vi "Conversor_4dados.vi"(2 "subarray":u8[](array[numeric])) -> (3 "ROCOF":sgl format="%_8g", 4 "Frequência":sgl format="%_8g", 5 "Ângulo":sgl format="%_8g", 6 "Módulo":sgl format="%_8g")   [LabVIEW 2018]
panel:
  out "sinal 4":bool
  out "sinal 3":bool
  out "sinal 2":bool
  out "sinal":bool
  # "Conversor de dados da serial - quadruplo"
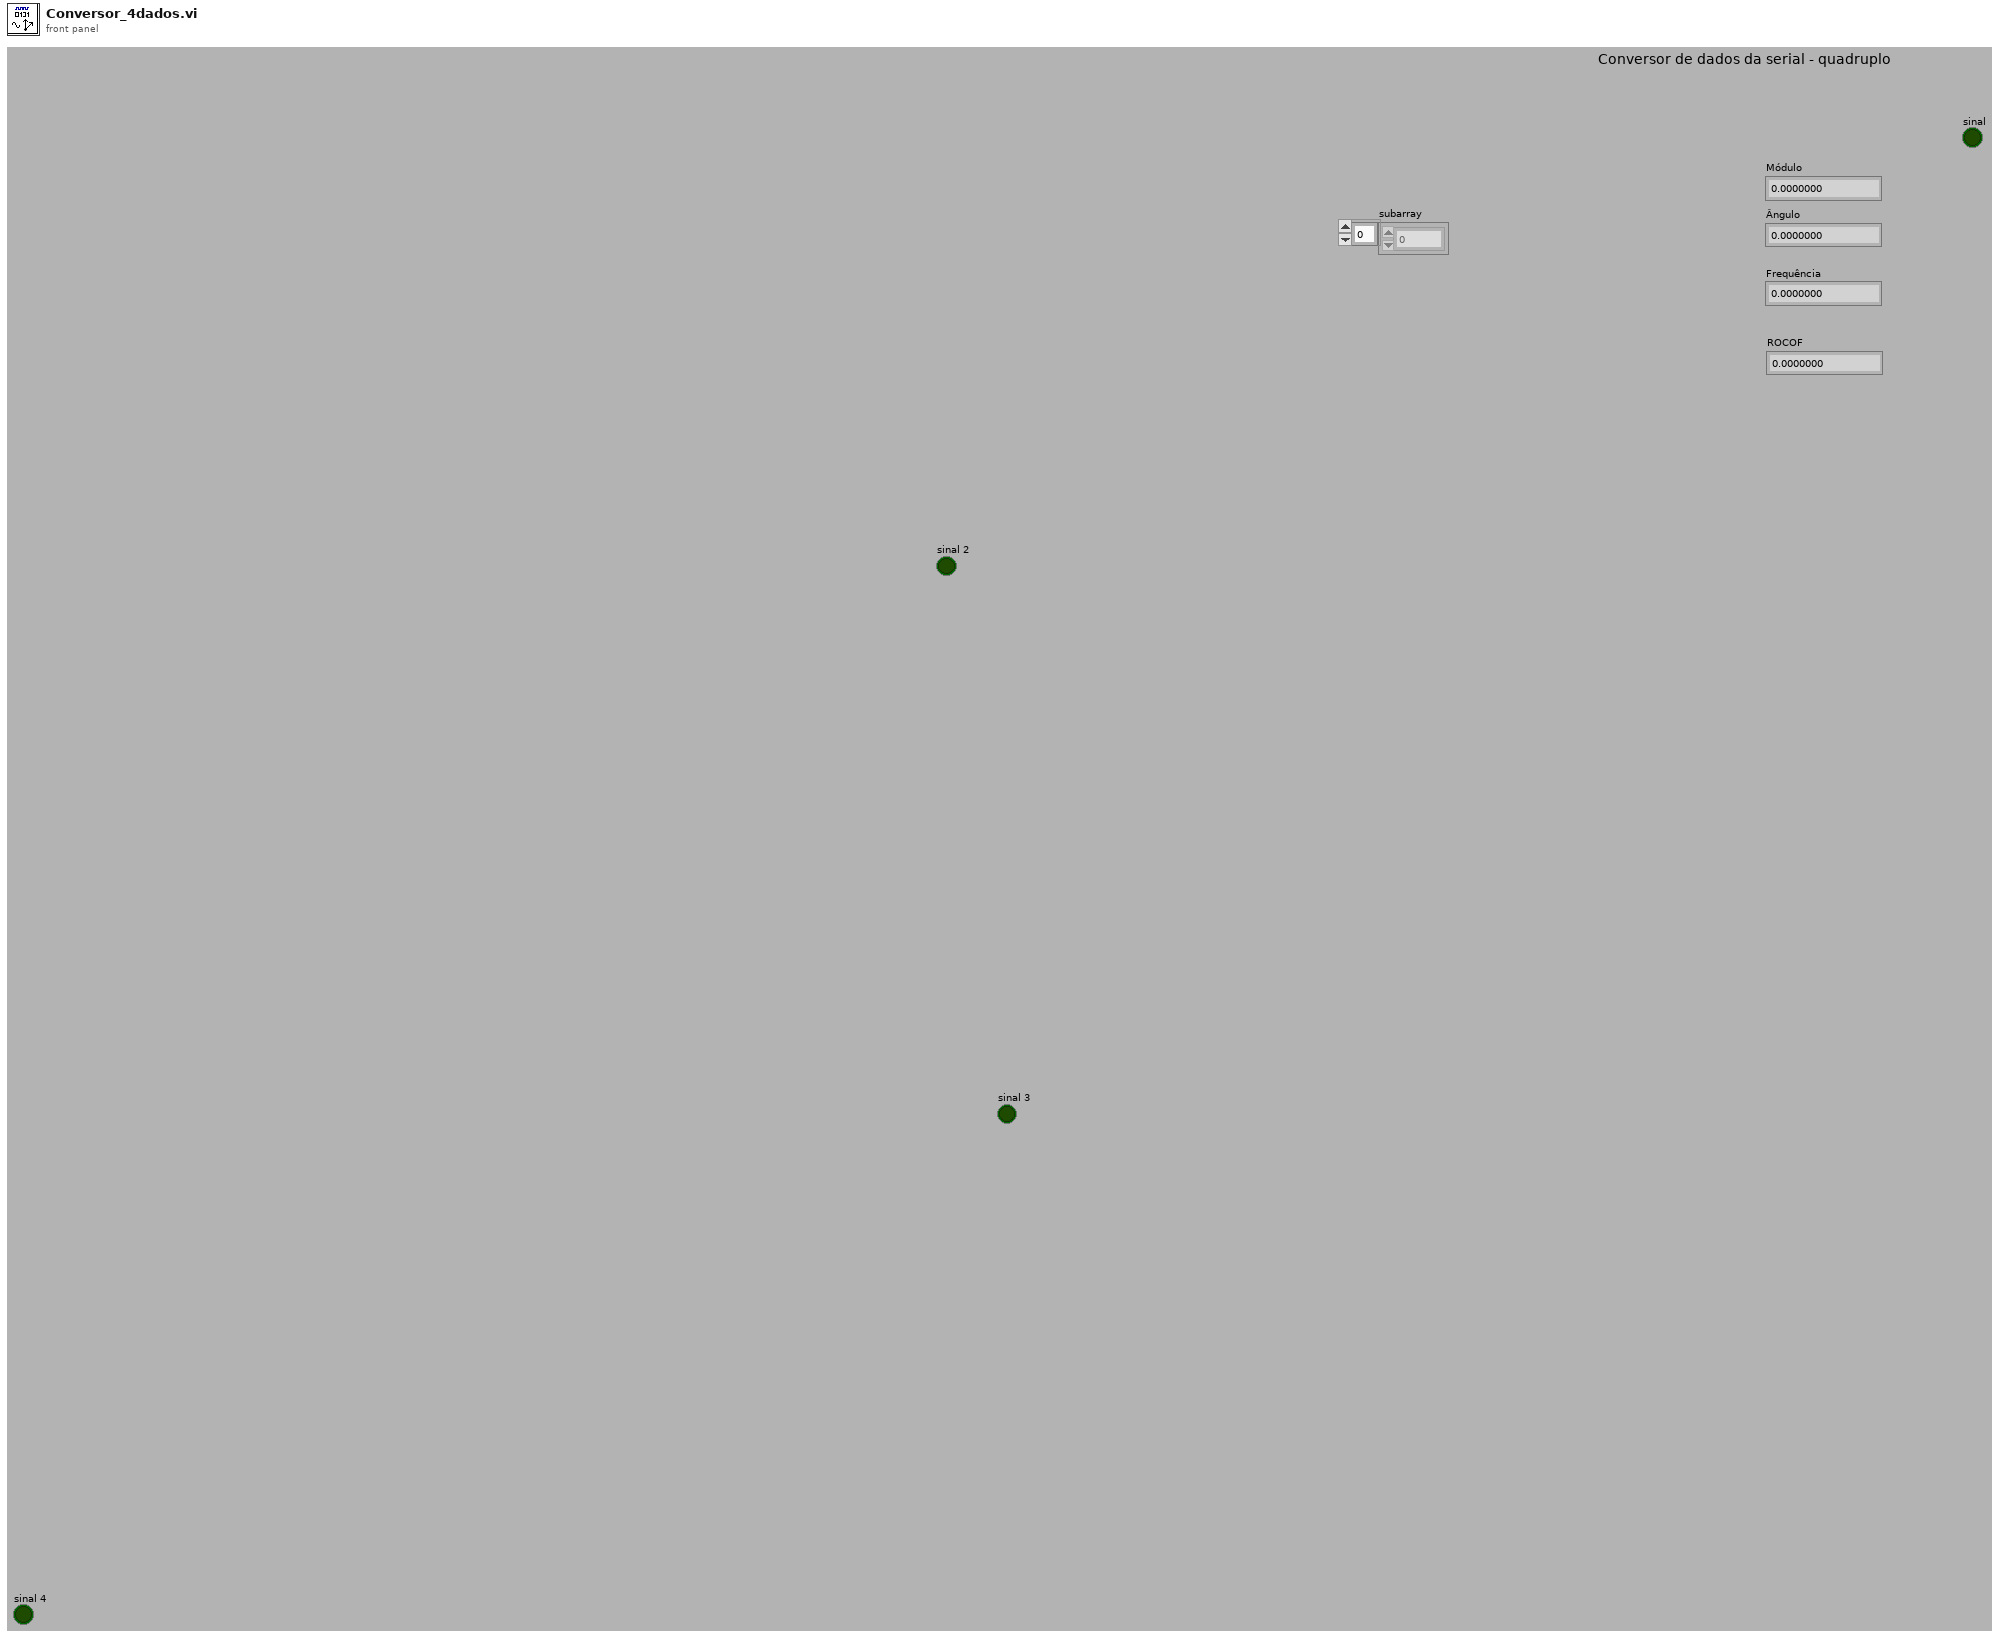
[diagram p1: front panel]
types:
  T1 = cluster{"[0]":u8, "[1]":u8, "[2]":u8, "[3]":u8, "[4]":u8, "[5]":u8, "[6]":u8, "[7]":u8, "[8]":u8}
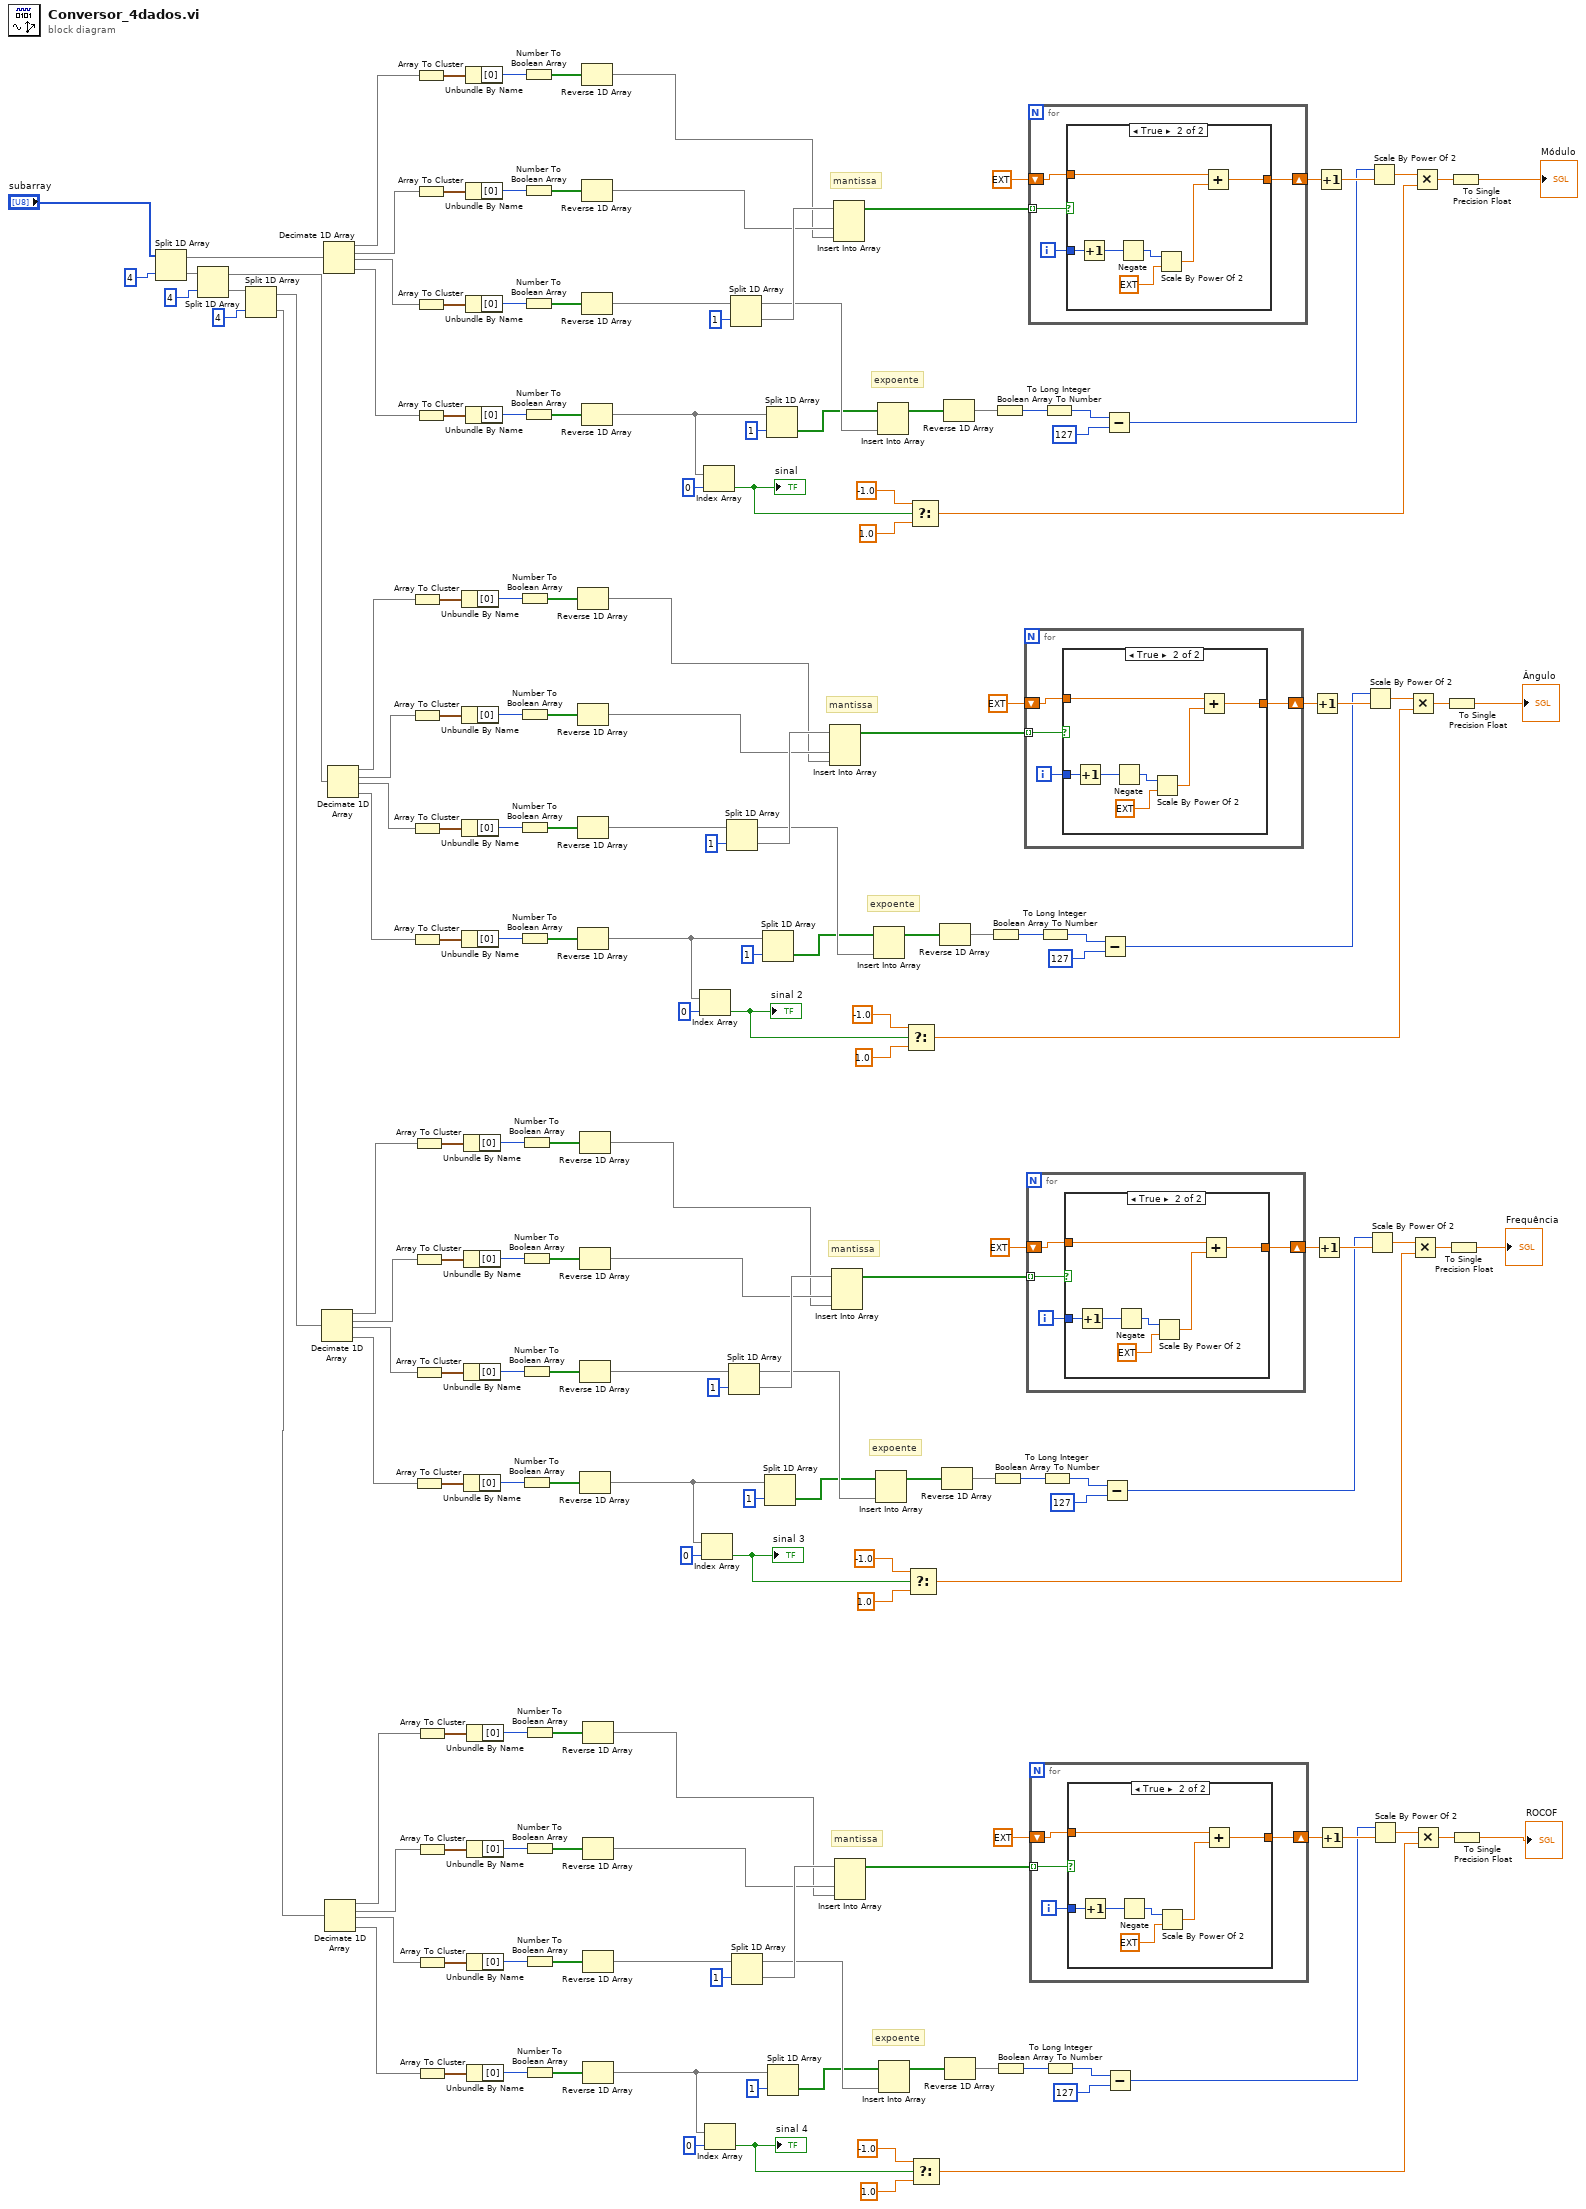
[diagram p0: block diagram]
diagram:
  # "expoente"
  # "mantissa"
  # "expoente"
  # "mantissa"
  # "expoente"
  # "mantissa"
  # "expoente"
  # "mantissa"
  n1 = Split 1D Array(array="subarray", index=4) -> (first subarray=w53:u8[], second subarray=w52:u8[])
  n2 = Split 1D Array(array=w52, index=4) -> (first subarray=w51:u8[], second subarray=w3:u8[])
  n3 = Split 1D Array(array=w3, index=4) -> (first subarray=w2:u8[], second subarray=w1:u8[])
  n4 = Decimate 1D Array(w2) -> (w88:u8[], w87:u8[], w86:u8[], w96:u8[])
  n5 = Decimate 1D Array(w53) -> (w174:u8[], w173:u8[], w172:u8[], w182:u8[])
  n6 = Decimate 1D Array(w1) -> (w39:u8[], w38:u8[], w37:u8[], w47:u8[])
  n7 = Decimate 1D Array(w51) -> (w131:u8[], w130:u8[], w129:u8[], w139:u8[])
  n8 = Array To Cluster(array=w131) -> (cluster=w133:T1)
  n9 = Array To Cluster(array=w130) -> (cluster=w135:T1)
  n10 = Array To Cluster(array=w129) -> (cluster=w137:T1)
  n11 = Array To Cluster(array=w139) -> (cluster=w138:T1)
  n12 = Array To Cluster(array=w88) -> (cluster=w90:T1)
  n13 = Array To Cluster(array=w87) -> (cluster=w92:T1)
  n14 = Array To Cluster(array=w86) -> (cluster=w94:T1)
  n15 = Array To Cluster(array=w96) -> (cluster=w95:T1)
  n16 = Array To Cluster(array=w174) -> (cluster=w176:T1)
  n17 = Array To Cluster(array=w173) -> (cluster=w178:T1)
  n18 = Array To Cluster(array=w172) -> (cluster=w180:T1)
  n19 = Array To Cluster(array=w182) -> (cluster=w181:T1)
  n20 = Array To Cluster(array=w39) -> (cluster=w41:T1)
  n21 = Array To Cluster(array=w38) -> (cluster=w43:T1)
  n22 = Array To Cluster(array=w37) -> (cluster=w45:T1)
  n23 = Array To Cluster(array=w47) -> (cluster=w46:T1)
  n24 = Unbundle By Name(w133) -> ("[0]"=w132:u8)
  n25 = Unbundle By Name(w135) -> ("[0]"=w134:u8)
  n26 = Unbundle By Name(w137) -> ("[0]"=w136:u8)
  n27 = Unbundle By Name(w138) -> ("[0]"=w125:u8)
  n28 = Unbundle By Name(w90) -> ("[0]"=w89:u8)
  n29 = Unbundle By Name(w92) -> ("[0]"=w91:u8)
  n30 = Unbundle By Name(w94) -> ("[0]"=w93:u8)
  n31 = Unbundle By Name(w95) -> ("[0]"=w82:u8)
  n32 = Unbundle By Name(w176) -> ("[0]"=w175:u8)
  n33 = Unbundle By Name(w178) -> ("[0]"=w177:u8)
  n34 = Unbundle By Name(w180) -> ("[0]"=w179:u8)
  n35 = Unbundle By Name(w181) -> ("[0]"=w168:u8)
  n36 = Unbundle By Name(w41) -> ("[0]"=w40:u8)
  n37 = Unbundle By Name(w43) -> ("[0]"=w42:u8)
  n38 = Unbundle By Name(w45) -> ("[0]"=w44:u8)
  n39 = Unbundle By Name(w46) -> ("[0]"=w33:u8)
  n40 = Number To Boolean Array(number=w132) -> (Boolean array=w116:bool[])
  n41 = Number To Boolean Array(number=w134) -> (Boolean array=w117:bool[])
  n42 = Number To Boolean Array(number=w136) -> (Boolean array=w118:bool[])
  n43 = Number To Boolean Array(number=w125) -> (Boolean array=w121:bool[])
  n44 = Number To Boolean Array(number=w89) -> (Boolean array=w73:bool[])
  n45 = Number To Boolean Array(number=w91) -> (Boolean array=w74:bool[])
  n46 = Number To Boolean Array(number=w93) -> (Boolean array=w75:bool[])
  n47 = Number To Boolean Array(number=w82) -> (Boolean array=w78:bool[])
  n48 = Number To Boolean Array(number=w175) -> (Boolean array=w159:bool[])
  n49 = Number To Boolean Array(number=w177) -> (Boolean array=w160:bool[])
  n50 = Number To Boolean Array(number=w179) -> (Boolean array=w161:bool[])
  n51 = Number To Boolean Array(number=w168) -> (Boolean array=w164:bool[])
  n52 = Number To Boolean Array(number=w40) -> (Boolean array=w24:bool[])
  n53 = Number To Boolean Array(number=w42) -> (Boolean array=w25:bool[])
  n54 = Number To Boolean Array(number=w44) -> (Boolean array=w26:bool[])
  n55 = Number To Boolean Array(number=w33) -> (Boolean array=w29:bool[])
  n56 = Reverse 1D Array(array=w116) -> (reversed array=w122:bool[])
  n57 = Reverse 1D Array(array=w117) -> (reversed array=w123:bool[])
  n58 = Reverse 1D Array(array=w118) -> (reversed array=w126:bool[])
  n59 = Reverse 1D Array(array=w121) -> (reversed array=w119:bool[])
  n60 = Reverse 1D Array(array=w73) -> (reversed array=w79:bool[])
  n61 = Reverse 1D Array(array=w74) -> (reversed array=w80:bool[])
  n62 = Reverse 1D Array(array=w75) -> (reversed array=w83:bool[])
  n63 = Reverse 1D Array(array=w78) -> (reversed array=w76:bool[])
  n64 = Reverse 1D Array(array=w159) -> (reversed array=w165:bool[])
  n65 = Reverse 1D Array(array=w160) -> (reversed array=w166:bool[])
  n66 = Reverse 1D Array(array=w161) -> (reversed array=w169:bool[])
  n67 = Reverse 1D Array(array=w164) -> (reversed array=w162:bool[])
  n68 = Reverse 1D Array(array=w24) -> (reversed array=w30:bool[])
  n69 = Reverse 1D Array(array=w25) -> (reversed array=w31:bool[])
  n70 = Reverse 1D Array(array=w26) -> (reversed array=w34:bool[])
  n71 = Reverse 1D Array(array=w29) -> (reversed array=w27:bool[])
  n72 = Index Array(array=w119, index=0) -> (element=w108:bool)
  "sinal 2" <- w108
  n73 = Index Array(array=w76, index=0) -> (element=w65:bool)
  "sinal 3" <- w65
  n74 = Index Array(array=w162, index=0) -> (element=w151:bool)
  "sinal" <- w151
  n75 = Index Array(array=w27, index=0) -> (element=w16:bool)
  "sinal 4" <- w16
  n76 = Split 1D Array(array=w126, index=1) -> (first subarray=w101:bool[], second subarray=w124:bool[])
  n77 = Split 1D Array(array=w83, index=1) -> (first subarray=w58:bool[], second subarray=w81:bool[])
  n78 = Split 1D Array(array=w169, index=1) -> (first subarray=w144:bool[], second subarray=w167:bool[])
  n79 = Split 1D Array(array=w34, index=1) -> (first subarray=w9:bool[], second subarray=w32:bool[])
  n80 = Split 1D Array(array=w119, index=1) -> (second subarray=w100:bool[])  [unwired: 1 out]
  n81 = Split 1D Array(array=w76, index=1) -> (second subarray=w57:bool[])  [unwired: 1 out]
  n82 = Split 1D Array(array=w162, index=1) -> (second subarray=w143:bool[])  [unwired: 1 out]
  n83 = Split 1D Array(array=w27, index=1) -> (second subarray=w8:bool[])  [unwired: 1 out]
  n84 = Insert Into Array(array=w124, new element #1=w123, new element #2=w122) -> (w102:bool[])  [unwired: 1 in]
  n85 = Insert Into Array(array=w81, new element #1=w80, new element #2=w79) -> (w59:bool[])  [unwired: 1 in]
  n86 = Insert Into Array(array=w167, new element #1=w166, new element #2=w165) -> (w145:bool[])  [unwired: 1 in]
  n87 = Insert Into Array(array=w32, new element #1=w31, new element #2=w30) -> (w10:bool[])  [unwired: 1 in]
  n88 = Insert Into Array(array=w100, new element=w101) -> (w99:bool[])  [unwired: 1 in]
  n89 = Insert Into Array(array=w57, new element=w58) -> (w56:bool[])  [unwired: 1 in]
  n90 = Insert Into Array(array=w143, new element=w144) -> (w142:bool[])  [unwired: 1 in]
  n91 = Insert Into Array(array=w8, new element=w9) -> (w7:bool[])  [unwired: 1 in]
  n92 = Select(t=-1.0, s=w108, f=1.0) -> (s? t:f=w104:dbl)
  n93 = Select(t=-1.0, s=w65, f=1.0) -> (s? t:f=w61:dbl)
  n94 = Select(t=-1.0, s=w151, f=1.0) -> (s? t:f=w147:dbl)
  n95 = Select(t=-1.0, s=w16, f=1.0) -> (s? t:f=w12:dbl)
  n96 = Reverse 1D Array(array=w99) -> (reversed array=w98:bool[])
  n97 = Reverse 1D Array(array=w56) -> (reversed array=w55:bool[])
  n98 = Reverse 1D Array(array=w142) -> (reversed array=w141:bool[])
  n99 = Reverse 1D Array(array=w7) -> (reversed array=w6:bool[])
  n100 = Boolean Array To Number(Boolean array=w98) -> (number=w112:u32)
  n101 = Boolean Array To Number(Boolean array=w55) -> (number=w69:u32)
  n102 = Boolean Array To Number(Boolean array=w141) -> (number=w155:u32)
  n103 = Boolean Array To Number(Boolean array=w6) -> (number=w20:u32)
  n104 = for {
    tunnel: w102 -> [w186] mode=indexing
    shift-right: [w184] -> w111
    shift-left: ext 0.0 -> [w183]
    i -> [w185]
    n105 = case shown="True" w186 {
      tunnel: w185 -> [_ w194]
      tunnel: [w187 w189] -> w184
      tunnel: w183 -> [w187 w188]
      frame False {
      }
      frame True {
        n106 = Increment(x=w194) -> (x+1=w193:i32)
        n107 = Negate(x=w193) -> (-x=w192:i32)
        n108 = Scale By Power Of 2(n=w192, x=ext 1.0) -> (x*2^n=w190:ext)
        n109 = Add(x=w188, y=w190) -> (x+y=w189:ext)
      }
    }
  }
  n110 = for {
    tunnel: w59 -> [w198] mode=indexing
    shift-right: [w196] -> w68
    shift-left: ext 0.0 -> [w195]
    i -> [w197]
    n111 = case shown="True" w198 {
      tunnel: w197 -> [_ w206]
      tunnel: [w199 w201] -> w196
      tunnel: w195 -> [w199 w200]
      frame False {
      }
      frame True {
        n112 = Increment(x=w206) -> (x+1=w205:i32)
        n113 = Negate(x=w205) -> (-x=w204:i32)
        n114 = Scale By Power Of 2(n=w204, x=ext 1.0) -> (x*2^n=w202:ext)
        n115 = Add(x=w200, y=w202) -> (x+y=w201:ext)
      }
    }
  }
  n116 = for {
    tunnel: w145 -> [w210] mode=indexing
    shift-right: [w208] -> w154
    shift-left: ext 0.0 -> [w207]
    i -> [w209]
    n117 = case shown="True" w210 {
      tunnel: w209 -> [_ w218]
      tunnel: [w211 w213] -> w208
      tunnel: w207 -> [w211 w212]
      frame False {
      }
      frame True {
        n118 = Increment(x=w218) -> (x+1=w217:i32)
        n119 = Negate(x=w217) -> (-x=w216:i32)
        n120 = Scale By Power Of 2(n=w216, x=ext 1.0) -> (x*2^n=w214:ext)
        n121 = Add(x=w212, y=w214) -> (x+y=w213:ext)
      }
    }
  }
  n122 = for {
    tunnel: w10 -> [w222] mode=indexing
    shift-right: [w220] -> w19
    shift-left: ext 0.0 -> [w219]
    i -> [w221]
    n123 = case shown="True" w222 {
      tunnel: w221 -> [_ w230]
      tunnel: [w223 w225] -> w220
      tunnel: w219 -> [w223 w224]
      frame False {
      }
      frame True {
        n124 = Increment(x=w230) -> (x+1=w229:i32)
        n125 = Negate(x=w229) -> (-x=w228:i32)
        n126 = Scale By Power Of 2(n=w228, x=ext 1.0) -> (x*2^n=w226:ext)
        n127 = Add(x=w224, y=w226) -> (x+y=w225:ext)
      }
    }
  }
  n128 = To Long Integer(number=w112) -> (32bit integer=w114:i32)
  n129 = To Long Integer(number=w69) -> (32bit integer=w71:i32)
  n130 = To Long Integer(number=w155) -> (32bit integer=w157:i32)
  n131 = To Long Integer(number=w20) -> (32bit integer=w22:i32)
  n132 = Subtract(x=w114, y=127) -> (x-y=w109:i32)
  n133 = Subtract(x=w71, y=127) -> (x-y=w66:i32)
  n134 = Subtract(x=w157, y=127) -> (x-y=w152:i32)
  n135 = Subtract(x=w22, y=127) -> (x-y=w17:i32)
  n136 = Increment(x=w111) -> (x+1=w110:ext)
  n137 = Increment(x=w68) -> (x+1=w67:ext)
  n138 = Increment(x=w154) -> (x+1=w153:ext)
  n139 = Increment(x=w19) -> (x+1=w18:ext)
  n140 = Scale By Power Of 2(n=w109, x=w110) -> (x*2^n=w105:ext)
  n141 = Scale By Power Of 2(n=w66, x=w67) -> (x*2^n=w62:ext)
  n142 = Scale By Power Of 2(n=w152, x=w153) -> (x*2^n=w148:ext)
  n143 = Scale By Power Of 2(n=w17, x=w18) -> (x*2^n=w13:ext)
  n144 = Multiply(x=w105, y=w104) -> (x*y=w103:ext)
  n145 = Multiply(x=w62, y=w61) -> (x*y=w60:ext)
  n146 = Multiply(x=w148, y=w147) -> (x*y=w146:ext)
  n147 = Multiply(x=w13, y=w12) -> (x*y=w11:ext)
  n148 = To Single Precision Float(number=w103) -> (single precision float=→"Ângulo":sgl)
  n149 = To Single Precision Float(number=w60) -> (single precision float=→"Frequência":sgl)
  n150 = To Single Precision Float(number=w146) -> (single precision float=→"Módulo":sgl)
  n151 = To Single Precision Float(number=w11) -> (single precision float=→"ROCOF":sgl)
